vi "资讯重打标签.vi"(7 "DBSet":T1, 8 "print path local":bool=TRUE, 9 "PN":string="L99QF015-SD-R", 10 "PRINT":refnum<k24>, 11 "SN":refnum<k24>) -> (1 "PrintMsg":string)   [LabVIEW 2011]
uses:
  Data/ClassLibraryMisWebservice.dll
panel:
  out "SN输入 2":string="1904051355/Z00A2R1647S000127"
  in  "制程条码":bool
  out "queried PN":string="L56QF026-SD-R"
  out "printPath":string
  in  "重打数目":i32=1
  in  "SN输入":string="1904051355/Z00A2R1647S000127"
  # "重打方法：\n第一步. 选择重打的数量\n第二步. 在SN输入处扫描条码"
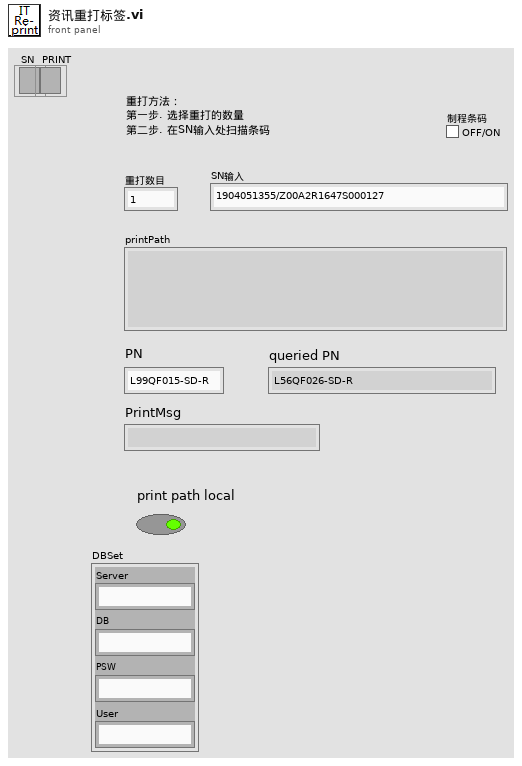
[diagram p1: front panel]
types:
  T1 = cluster{"Server":string, "DB":string, "PSW":string, "User":string}
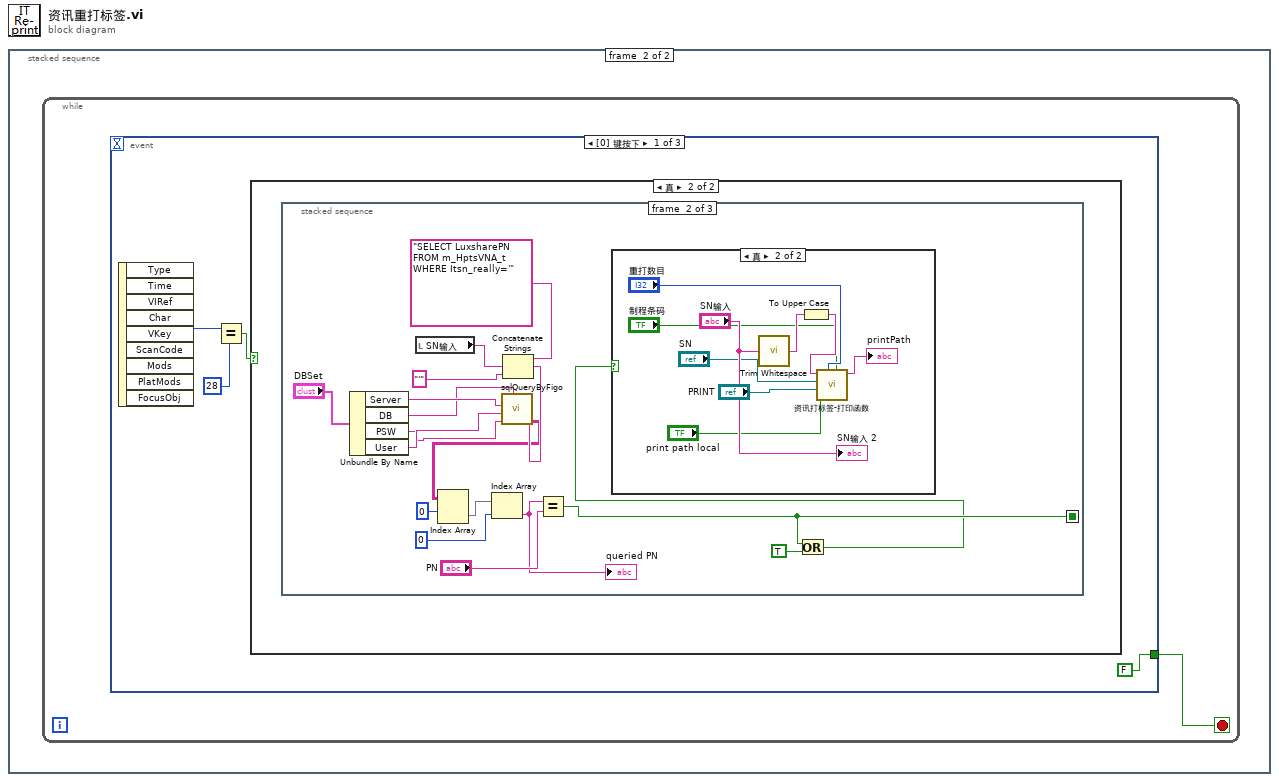
[diagram p0: block diagram]
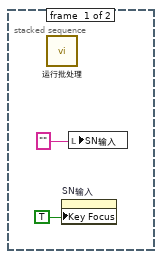
[diagram p2: hidden frame]
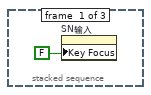
[diagram p4: hidden frame]
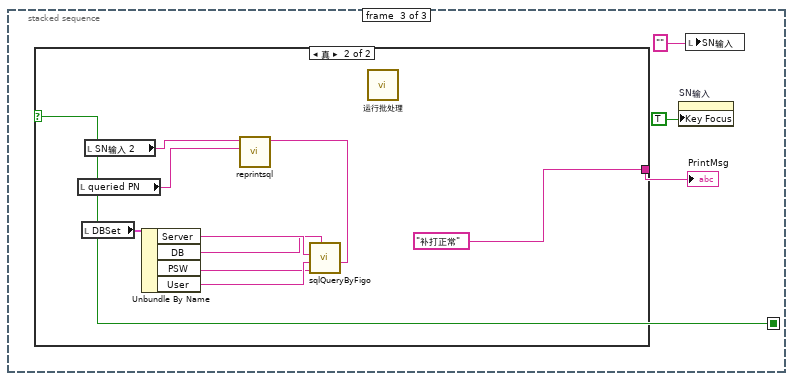
[diagram p6: hidden frame]
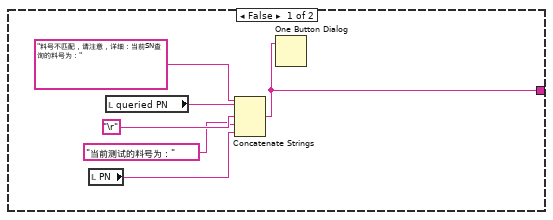
[diagram p7: hidden frame]
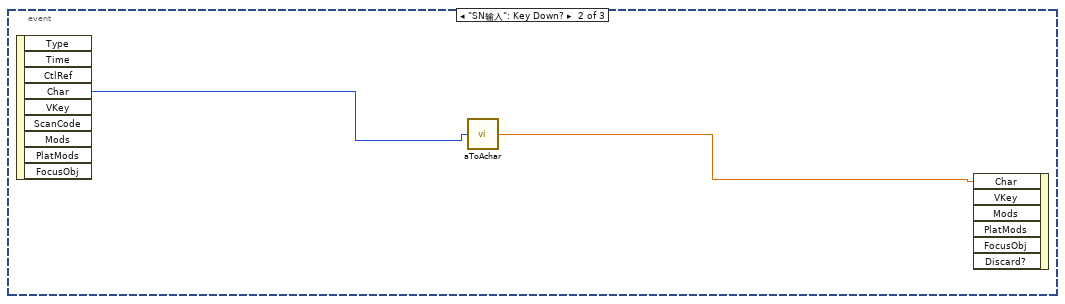
[diagram p8: hidden frame]
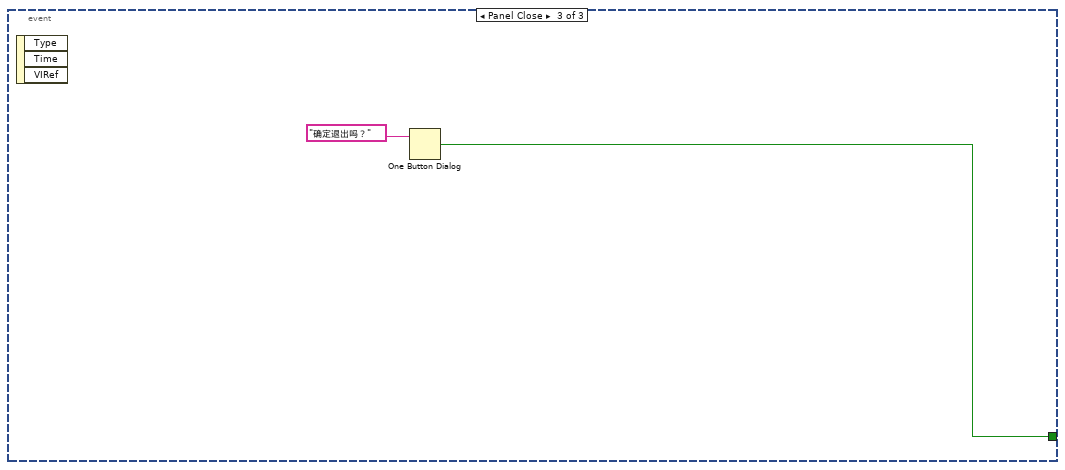
[diagram p9: hidden frame]
diagram:
  n1 = stacked-sequence {
    frame #0 {
      n2 = call "运行批处理.vi"() -> ()  [unwired: 12 in]
      n3 = property on="SN输入" class="Str"("Key Focus"=TRUE ("键选中")) -> ()  [unwired: 2 in, 2 out]
      n4 = local write "SN输入"("") -> ()
    }
    frame #1 {
      n5 = while {
        stop <- w3 stop-if-true
        n6 = event shown="[0] 键按下" {
          selector: _ -> [_ _ _]
          dyn-events: _ -> [_ _ _]
          timeout: _ -> [_ _ _]
          tunnel: [FALSE _ w57] -> w3
          event Key Down {
            n7 = event-data() -> ("ScanCode"=w7:i16)  [unwired: 1 in, 8 out]
            n8 = Equal?(x=w7, y=i16 28) -> (x = y?=w5:bool)
            n9 = case shown="真" w5 {
              frame False {
              }
              frame True {
                n10 = stacked-sequence {
                  seq-local: [_ w16 _] -> [_ _ w37]
                  frame #0 {
                    n11 = property on="SN输入" class="Str"("Key Focus"=FALSE ("键选中")) -> ()  [unwired: 2 in, 2 out]
                  }
                  frame #1 {
                    n12 = Unbundle By Name("DBSet") -> ("Server"=w12:string, "DB"=w9:string, "PSW"=w10:string, "User"=w11:string)
                    n13 = local read "SN输入"() -> (w24:string)
                    n14 = Concatenate Strings("SELECT LuxsharePN FROM m_HptsVNA_t WHERE Itsn_really='" ("字符串"), w24, "'" ("字符串")) -> (w23:string)
                    n15 = call "sqlQueryByFigo.vi"("SQL"=w23, "DATABASE"=w9, "password"=w10, "user id"=w11, "Server"=w12) -> ("查询数据"=w22:string[][])  [unwired: 5 in, 1 out]
                    n16 = Index Array(array=w22, index (row)=0 ("索引 (行)")) -> (element=w20:string[])  [unwired: 1 in]
                    n17 = Index Array(array=w20, index=0 ("索引")) -> (element=w17:string)
                    "queried PN" <- w17
                    n18 = Equal?(x=w17, y="PN") -> (x = y?=w16:bool)
                    n19 = Or(x=w16, y=TRUE) -> (x .or. y?=w14:bool)
                    n20 = case shown="真" w14 {
                      frame False {
                      }
                      frame True {
                        n21 = call <vilib>:"Trim Whitespace.vi"("string"="SN输入") -> ("trimmed string"=w31:string)  [unwired: 1 in]
                        n22 = To Upper Case(1:w31) -> (0:w30:string)
                        n23 = call "资讯打标签-打印函数.vi"("条码类型"="制程条码", "label num"="重打数目", "print path local"="print path local", "PRINT"="PRINT", "SN"="SN", "SN输入"=w30) -> ("printPath"=→"printPath":string)  [unwired: 4 in, 1 out]
                        "SN输入 2" <- "SN输入"
                      }
                    }
                  }
                  frame #2 {
                    n24 = case shown="真" w37 {
                      tunnel: [w40 "补打正常"] -> w36
                      frame False {
                        n25 = local read "PN"() -> (w41:string)
                        n26 = local read "queried PN"() -> (w44:string)
                        n27 = Concatenate Strings("料号不匹配，请注意，详细：当前SN查询的料号为：" ("字符串"), w44, "\r", "当前测试的料号为：" ("字符串"), w41) -> (w40:string)
                        n28 = One Button Dialog(message=w40) -> ()  [unwired: 1 in, 1 out]
                      }
                      frame True {
                        n29 = local read "queried PN"() -> (w51:string)
                        n30 = local read "DBSet"() -> (w50:T1)
                        n31 = local read "SN输入 2"() -> (w53:string)
                        n32 = Unbundle By Name(w50) -> ("Server"=w49:string, "DB"=w46:string, "PSW"=w47:string, "User"=w48:string)
                        n33 = call "reprintsql.vi"("pn"=w51, "sn"=w53) -> ("exec sql"=w52:string)  [unwired: 9 in]
                        n34 = call "sqlQueryByFigo.vi"("SQL"=w52, "DATABASE"=w46, "password"=w47, "user id"=w48, "Server"=w49) -> ()  [unwired: 5 in, 2 out]
                        n35 = call "运行批处理.vi"() -> ()  [unwired: 12 in]
                      }
                    }
                    "PrintMsg" <- w36
                    n36 = property on="SN输入" class="Str"("Key Focus"=TRUE ("键选中")) -> ()  [unwired: 2 in, 2 out]
                    n37 = local write "SN输入"("") -> ()
                  }
                }
              }
            }
          }
          event "SN输入": Key Down? {
            n38 = event-data() -> ("Char"=w56:i16)  [unwired: 1 in, 8 out]
            n39 = call "aToAchar.vi"("old char"=w56) -> ("new char"=w55:dbl)
            n40 = event-data("Char"=w55) -> ()  [unwired: 6 in, 1 out]
          }
          event Panel Close {
            n41 = event-data() -> ()  [unwired: 1 in, 3 out]
            n42 = One Button Dialog(message="确定退出吗？" ("消息")) -> (true=w57:bool)  [unwired: 1 in]
          }
        }
      }
    }
  }
